vi "BNO055 loop.vi"(8 "error in (no error)":errorcluster) -> ()   [LabVIEW 2019]
uses:
  Ver.2/BNO055 gyro 3axis.ctl
  <vilib>/Platform/TimedLoop/XDataNode/timing_clust.ctl
  <vilib>/Platform/TimedLoop/XDataNode/nitl_modes.ctl
  <vilib>/Platform/TimedLoop/XDataNode/wakeup.ctl
  <vilib>/platform/TimedLoop/XDataNode/XDataNode.xnode
  <vilib>/Platform/TimedLoop/XDataNode/XDNodeRunTimeDep.lvlib
panel:
  out "output cluster":T1
  out "error out 2":errorcluster
  out "error out":errorcluster
  in  "value":bool
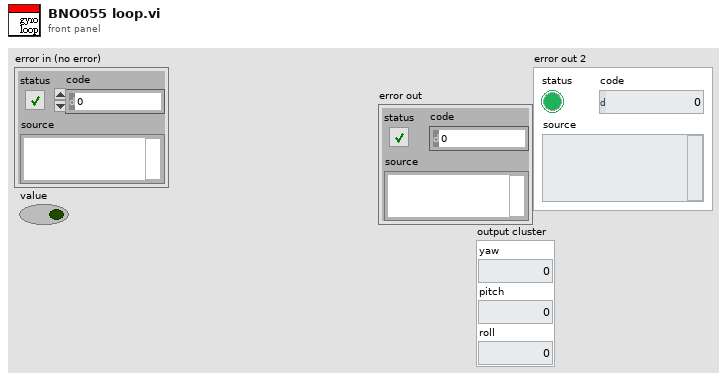
[diagram p1: front panel]
types:
  T1 = typedef "BNO055 gyro 3axis.ctl" = cluster{"yaw":dbl, "pitch":dbl, "roll":dbl}
  T2 = typedef "XDNodeRunTimeDep.lvlib/timing_clust.ctl" = cluster{"Expected End [f-1]":u64, "Actual End [f-1]":u64, "Finished Late? [f-1]":bool, "Expected End [i-1]":u64, "Actual End [i-1]":u64, "Finished Late? [i-1]":bool, "Expected Start [i]":u64, "Actual Start [i]":u64, "Expected Start [f]":u64, "Actual Start [f]":u64, "Source Name":string, "Structure Name":string, "Period":i64, "Deadline":i64, "Offset":i64, "Start":i64, "Priority":i32, "Timeout":i32, "Mode":T3, "Wakeup Reason":T4, "Error":errorcluster, "Source Type":string, "Secondary Source Type":string, "Global End Time":u64, "Global Start Time":u64, "Frame Duration":u64, "Iteration Duration":u64, "Assigned CPU":i32, "I/O Scan Engine Mode":u32}
  T3 = typedef "XDNodeRunTimeDep.lvlib/nitl_modes.ctl" = enum32{"No Change", "Process missed periods, maintain original phase", "Discard missed periods, maintain original phase", "Process missed periods, ignore original phase", "Discard missed periods, ignore original phase"}
  T4 = typedef "XDNodeRunTimeDep.lvlib/wakeup.ctl" = enum32{"Normal", "Aborted", "Asynchronous wakeup", "Timing source error", "Timed loop error", "Timeout"}
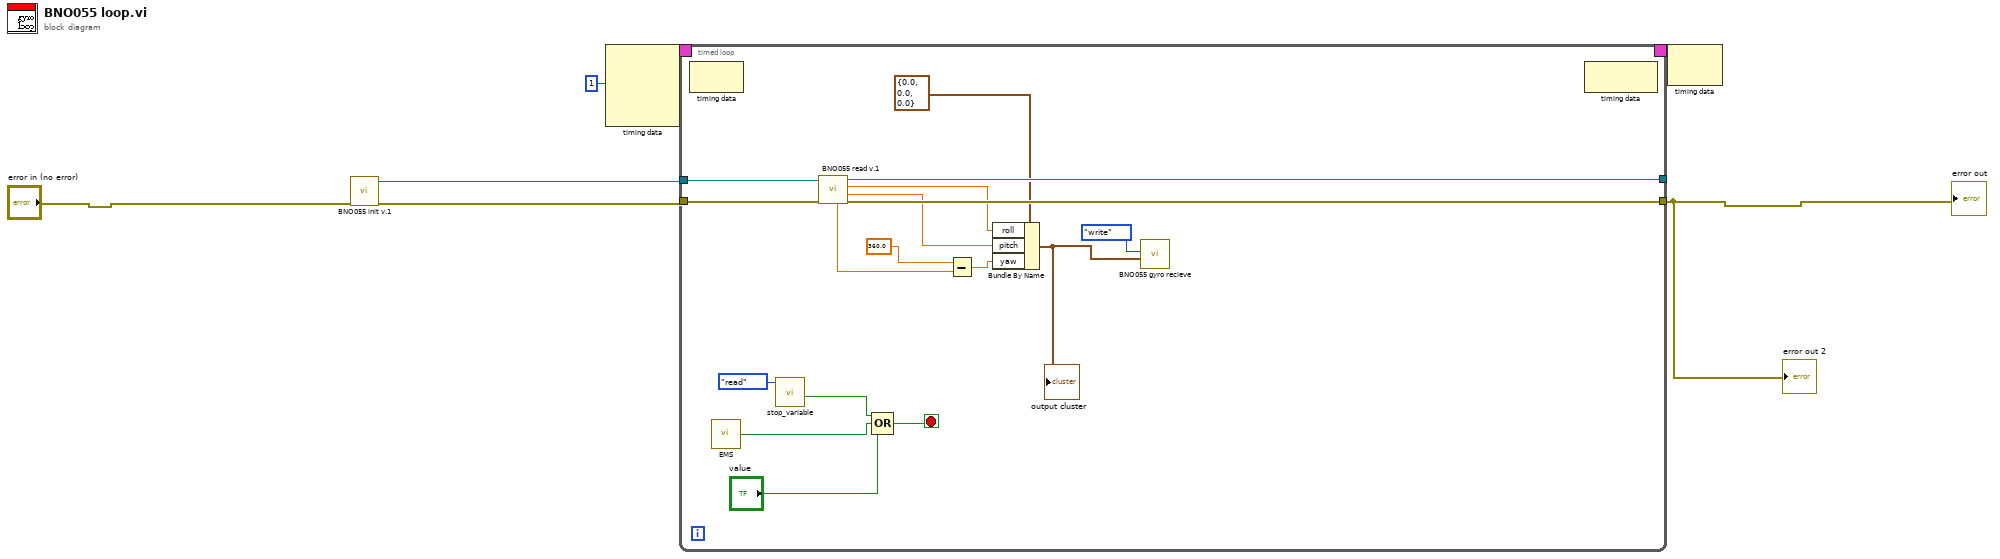
[diagram p0: block diagram]
diagram:
  n1 = call "BNO055 init v.1.vi"("error in (no error)"="error in (no error)") -> ("error out"=w7:errorcluster, "I2C out"=w6:refnum<class "I2C.lvclass">)  [unwired: 9 in]
  n2 = node-c288(i64 1 ("Period")) -> (w5:T2)  [unwired: 3 in]
  n3 = timed-loop {
    tunnel: w6 -> [w23]
    tunnel: w7 -> [w22]
    tunnel: [w24] -> _
    tunnel: [w21] -> w1
    timing: w5 -> [_]
    timing-out: [_] -> w4
    stop <- w19 stop-if-true
    n4 = node-c288() -> ()  [unwired: 1 in, 1 out]
    n5 = call "EMS.vi"() -> ("A/DIO4 (Pin 19)"=w17:bool)
    n6 = call "stop_variable.vi"("Enum"=enum16{"read", "write"}."read") -> ("read"=w18:bool)  [unwired: 10 in]
    n7 = call "BNO055 read v.1.vi"("error in (no error)"=w22, "I2C in"=w23) -> ("error out"=w21:errorcluster, "pitch"=w11:dbl, "roll"=w10:dbl, "I2C out"=w24:refnum<class "I2C.lvclass">, "yaw"=w9:dbl)  [unwired: 5 in]
    n8 = Compound Arithmetic op=OR(w18, w17, "value") -> (w19:bool)
    n9 = Subtract(x=360.0 ("y"), y=w9) -> (x-y=w14:dbl)
    n10 = Bundle By Name(cluster=T1 {"yaw"=0.0, "pitch"=0.0, "roll"=0.0} ("gyro"), "roll"=w10, "pitch"=w11, "yaw"=w14) -> (w12:T1)
    "output cluster" <- w12
    n11 = call "BNO055 gyro recieve.vi"("Write"=w12, "Enum"=enum16{"read", "write"}."write") -> ()  [unwired: 9 in, 1 out]
    n12 = node-c288() -> ()  [unwired: 1 in, 1 out]
  }
  "error out" <- w1
  "error out 2" <- w1
  n13 = node-c288(w4) -> ()  [unwired: 1 out]
